vi "Execute.vi"(8 "error in (no error)":errorcluster, 10 "Abstract Consumer in":refnum<class "Abstract Consumer.lvclass">, 11 "Test Message in":refnum<class "Test Message.lvclass">) -> (0 "error out":errorcluster, 1 "Abstract Response out":refnum<class "Abstract Response Message.lvclass">, 2 "Abstract Consumer out":refnum<class "Abstract Consumer.lvclass">, 3 "Test Message out":refnum<class "Test Message.lvclass">, 4 "Stop?":bool)   [LabVIEW 2017, in "Test Message.lvclass"]
uses:
  Test Message.lvclass
  Consumer/Abstract Consumer/Abstract Consumer.lvclass
  Message/Abstract Response Message/Abstract Response Message.lvclass
  Message List Action.ctl
  Message String Action.ctl
  Test Message.lvclass/Test Message.ctl
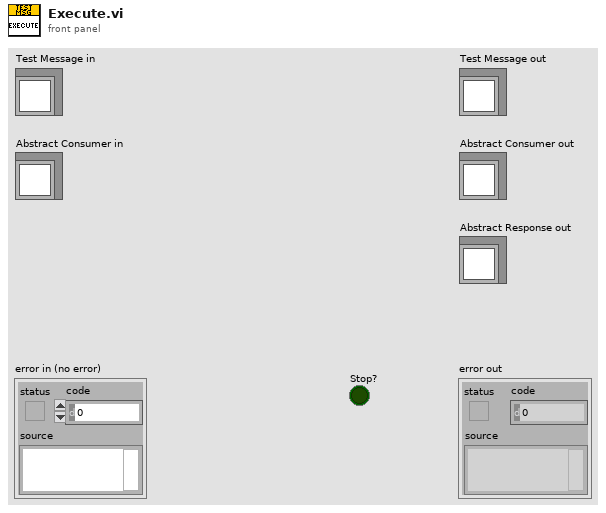
[diagram p1: front panel]
types:
  T1 = typedef "Message String Action.ctl" = enum16{"Get String", "Set String", "Reset"}
  T2 = typedef "Message List Action.ctl" = enum16{"Get", "Add", "Reset"}
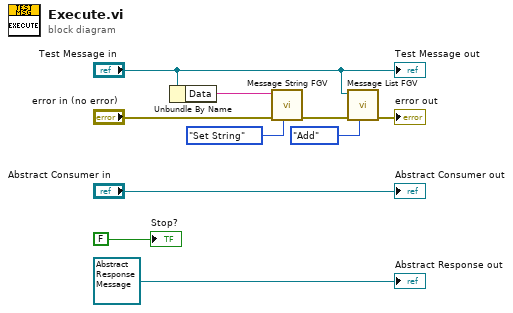
[diagram p0: block diagram]
diagram:
  n1 = Unbundle By Name("Test Message in") -> ("Data"=w1:string)
  n2 = call "Message String FGV.vi"("Action"=Message_String_Action."Set String", "error in (no error)"="error in (no error)", "Message String"=w1) -> ("error out"=w2:errorcluster)  [unwired: 7 in, 1 out]
  n3 = call "Message List FGV.vi"("Action (Get)"=Message_List_Action."Add", "error in (no error)"=w2, "Message Object"="Test Message in") -> ("error out"=→"error out":errorcluster)  [unwired: 7 in, 1 out]
  "Test Message out" <- "Test Message in"
  "Abstract Consumer out" <- "Abstract Consumer in"
  "Stop?" <- FALSE ("Stop?")
  "Abstract Response out" <- refnum<class "Abstract Response Message.lvclass"> refnum ("Abstract Response out")
